vi "Format Chuck-Slot.vi"(8 "error in":errorcluster, 9 "Slot":i32, 10 "Chuck":i32, 11 "Console Log in":refnum<class "Console Log.lvclass">) -> (0 "error out":errorcluster, 2 "Formatted Chuck/Slot":string, 3 "Console Log out":refnum<class "Console Log.lvclass">)   [LabVIEW 2011, in "Console Log.lvclass"]
uses:
  Console Log.lvclass
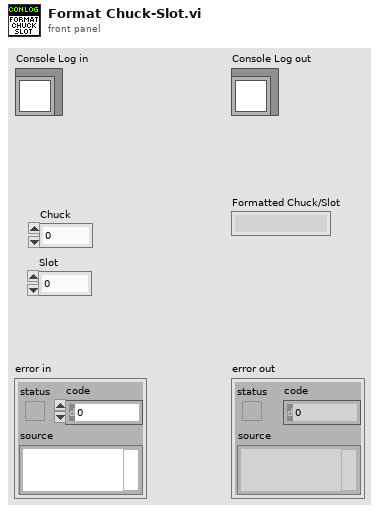
[diagram p1: front panel]
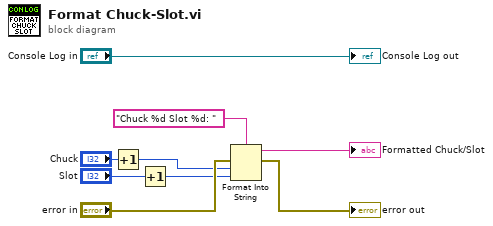
[diagram p0: block diagram]
diagram:
  n1 = Increment(x="Chuck") -> (x+1=w3:i32)
  n2 = Increment(x="Slot") -> (x+1=w1:i32)
  n3 = Format Into String(format string="Chuck %d Slot %d: ", error in="error in", w3, w1) -> (resulting string=→"Formatted Chuck/Slot":string, error out=→"error out":errorcluster)  [unwired: 1 in]
  "Console Log out" <- "Console Log in"
